vi "Leaktest Data to File v10.vi"(0 "Elapsed Sec":u32, 1 "Dir Path":path, 2 "Fallback Location":T3={"Log directory type"=1, "Rel Log Path"="LeakTemp"} {"Log directory type" items=["User Home"=0, "User Desktop"=1, "User Documents"=2, "User Application Data"=3, "User Preferences"=4, "User Temporary"=5, "Public Documents"=6, "Public Application Data"=7, "Public Preferences"=8, "Public Cache"=13, "System Core Libraries"=9, "System Installed Libraries"=10, "Application Files"=11, "Boot Volume Root"=12]}, 3 "File Name":string, 4 "Time Fmt":enum16{"H:M:S", "Days", "Secs"}(ring)=enum."Days", 5 "Leaktest Data":T1 {"Diff H2O" format="%.2g"; "Ref PSIA" format="%.2g"; "Fill PSIA" format="%.2g"; "Heat %" format="%.2g"; "Room dC" format="%.2g"; "Encl 1 dC" format="%.2g"}, 9 "precision":i16=3, 11 "error in":errorcluster, 12 "Header":string[](array[string])=["days.00000", "Fill PSIA", "Ref PSIA", "Diff \"H2O", "Encl degC", "Room degC", "Heater %"], 14 "Tester":string) -> (15 "error out":errorcluster)   [LabVIEW 2020]
uses:
  System Directory Type.ctl
panel:
  # "Dir Path, if valid, will be used in preference to local Windows File Location"
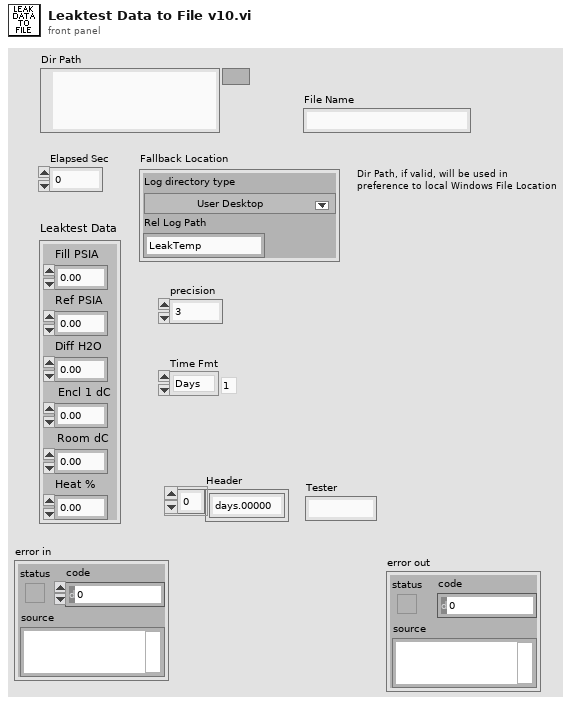
[diagram p1: front panel]
types:
  T1 = cluster{"Fill PSIA":dbl, "Ref PSIA":dbl, "Diff H2O":dbl, "Encl 1 dC":dbl, "Room dC ":dbl, "Heat %":dbl}
  T2 = typedef "System Directory Type.ctl" = i32
  T3 = cluster{"Log directory type":T2, "Rel Log Path":string}
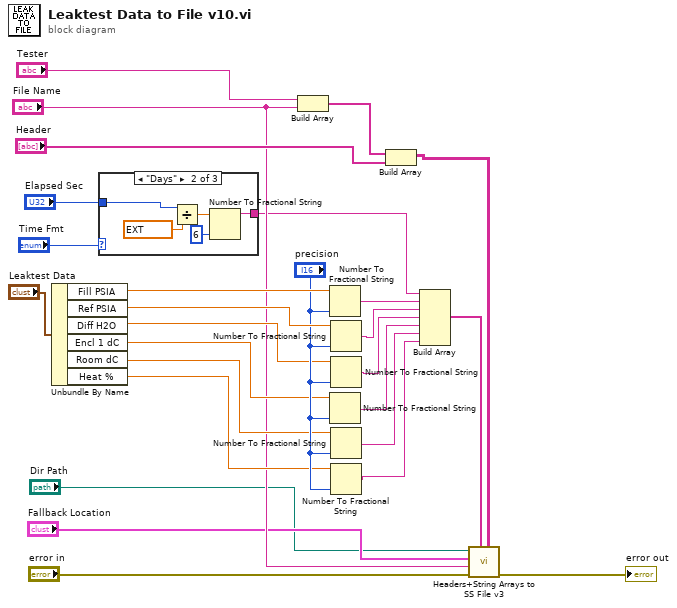
[diagram p0: block diagram]
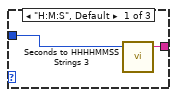
[diagram p2: hidden frame]
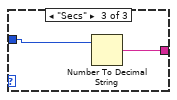
[diagram p3: hidden frame]
diagram:
  n1 = Unbundle By Name("Leaktest Data") -> ("Fill PSIA"=w20:dbl, "Ref PSIA"=w19:dbl, "Diff H2O"=w16:dbl, "Encl 1 dC"=w15:dbl, "Room dC"=w14:dbl, "Heat %"=w13:dbl)
  n2 = case shown="\"Days\"" "Time Fmt" {
    tunnel: [w29 w33 w35] -> w7
    tunnel: "Elapsed Sec" -> [w28 w31 w36]
    frame "H:M:S", Default {
      n3 = call "Seconds to HHHHMMSS Strings 3.vi"("Seconds"=w28) -> ("HHHH:MM:SS"=w29:string)  [unwired: 3 in, 1 out]
    }
    frame "Days" {
      n4 = Divide(x=w31, y=ext 86400.0) -> (x/y=w30:ext)
      n5 = Number To Fractional String(number=w30, precision (6)=i16 6) -> (F-format string=w33:string)  [unwired: 2 in]
    }
    frame "Secs" {
      n6 = Number To Decimal String(number=w36) -> (decimal integer string=w35:string)  [unwired: 1 in]
    }
  }
  n7 = Build Array("Tester", "File Name") -> (w24:string[])
  n8 = Number To Fractional String(number=w20, precision (6)="precision") -> (F-format string=w23:string)  [unwired: 2 in]
  n9 = Number To Fractional String(number=w15, precision (6)="precision") -> (F-format string=w10:string)  [unwired: 2 in]
  n10 = Number To Fractional String(number=w19, precision (6)="precision") -> (F-format string=w22:string)  [unwired: 2 in]
  n11 = Number To Fractional String(number=w16, precision (6)="precision") -> (F-format string=w18:string)  [unwired: 2 in]
  n12 = Number To Fractional String(number=w14, precision (6)="precision") -> (F-format string=w9:string)  [unwired: 2 in]
  n13 = Number To Fractional String(number=w13, precision (6)="precision") -> (F-format string=w8:string)  [unwired: 2 in]
  n14 = Build Array(w24, "Header") -> (w3:string[][])
  n15 = Build Array(w7, w23, w22, w18, w10, w9, w8) -> (w4:string[])
  n16 = call "Headers+String Arrays to SS File v3.vi"("Header"=w3, "1d Data String Array"=w4, "error in"="error in", "File Name"="File Name", "File Location"="Fallback Location", "Dir Path"="Dir Path") -> ("error out"=→"error out":errorcluster)  [unwired: 4 in, 1 out]
